vi "Set Buffer Filling Mode.vi"(0 "VISA resource name":refnum<visa-resource-name>, 5 "Buffer Name (defbuffer1)":string="defbuffer1", 7 "Fill Type":u16(ring) items=["Continuous", "Once"], 11 "error in (no error)":errorcluster) -> (4 "VISA resource name out":refnum<visa-resource-name>, 15 "error out":errorcluster)   [LabVIEW 2016, in "Keithley DMM7510.lvlib"]
doc: "This VI determines if a reading buffer is filled continuously or is filled once and stops."
uses:
  Keithley DMM7510.lvlib
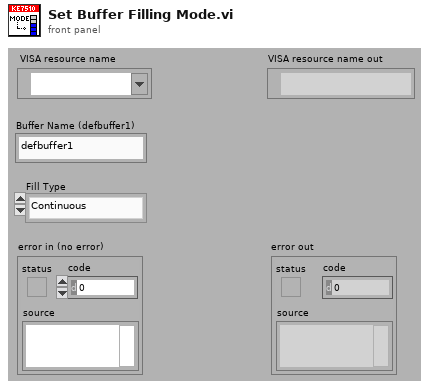
[diagram p1: front panel]
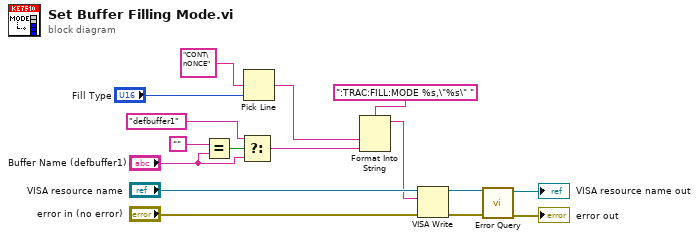
[diagram p0: block diagram]
diagram:
  n1 = Equal?(x="", y="Buffer Name (defbuffer1)") -> (x = y?=w13:bool)
  n2 = Select(t="defbuffer1", s=w13, f="Buffer Name (defbuffer1)") -> (s? t:f=w1:string)
  n3 = Pick Line(multi-line string="CONT\nONCE", line index="Fill Type") -> (output string=w3:string)  [unwired: 1 in]
  n4 = Format Into String(format string=":TRAC:FILL:MODE %s,\"%s\" " ("Fetch Measurement"), w3, w1) -> (resulting string=w2:string)  [unwired: 2 in, 1 out]
  n5 = VISA Write(VISA resource name="VISA resource name", write buffer=w2, error in (no error)="error in (no error)") -> (VISA resource name out=w8:refnum<visa-resource-name>, error out=w7:errorcluster)  [unwired: 1 out]
  n6 = call "Error Query.vi"("error in (no error)"=w7, "VISA resource name"=w8) -> ("error out"=→"error out":errorcluster, "VISA resource name out"=→"VISA resource name out":refnum<visa-resource-name>)  [unwired: 8 out]
